vi "Get Discovered Devices (SubVI).vi"(8 "error in":errorcluster, 9 "DeviceKey List":string[](array[string]), 10 "Master Count":i32, 11 "CmdLib In":refnum<k24>) -> (0 "error out":errorcluster, 1 "DeviceKey List Out":string[](array[string]), 2 "Device Array":T1(array[cluster]), 3 "CmdLib Out":refnum<k24>)   [LabVIEW 2017]
doc: "by Tanguy BOULARD"
uses:
  dll/CmdLib.dll
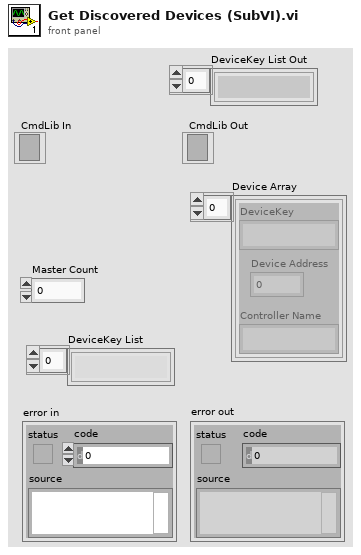
[diagram p1: front panel]
types:
  T1 = cluster{"DeviceKey":string, "Device Address":i32, "Controller Name":string}[]
  T2 = cluster{"DeviceKey Out":string, "Device Address Out":i32, "Controller Name":string}
  T3 = cluster{"DeviceKey Out":string, "Device Address Out":i32, "Controller Name":string}[]
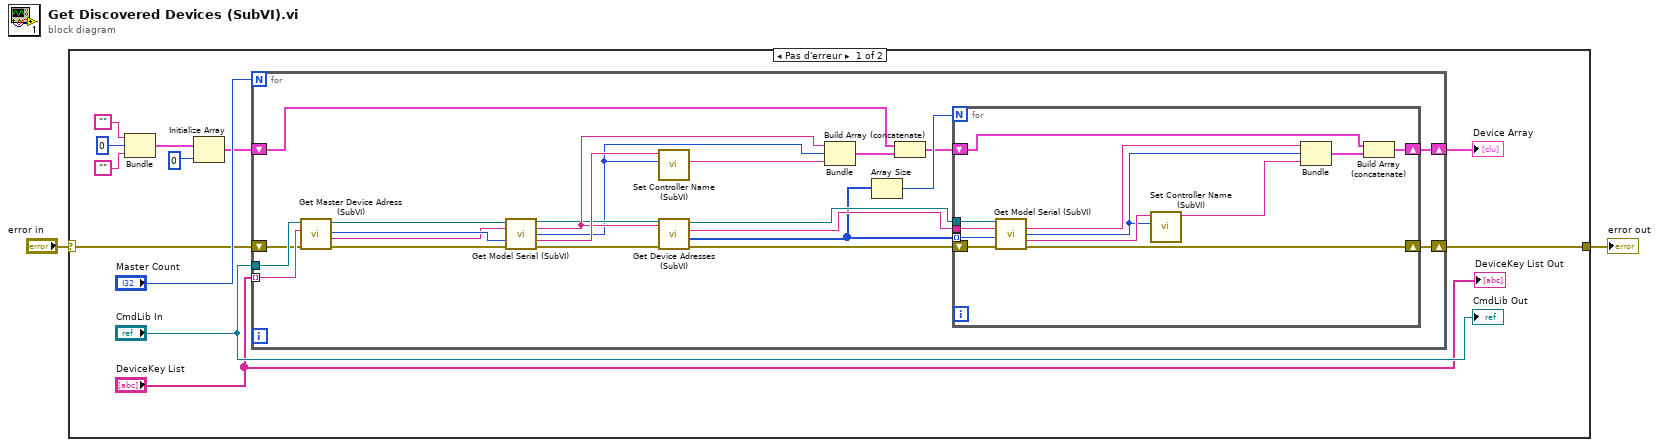
[diagram p0: block diagram]
diagram:
  n1 = case shown="Pas d'erreur" "error in" {
    selector: "error in" -> [w10 w50]
    tunnel: [w11 w50] -> w2
    frame No Error {
      n2 = Bundle("", 0, "") -> (w6:cluster{string, i32, string})  [unwired: 1 in]
      n3 = Initialize Array(w6, 0 ("dimension size")) -> (w4:cluster{string, i32, string}[])
      n4 = for {
        N: "Master Count" -> [_]
        tunnel: "CmdLib In" -> [w29]
        tunnel: "DeviceKey List" -> [w28] mode=indexing
        shift-right: [w26] -> w11
        shift-left: w10 -> [w27]
        shift-right: [w20] -> w3
        shift-left: w4 -> [w23]
        n5 = call "Get Master Device Adress (SubVI).vi"("entrée d'erreur (pas d'erreur)"=w27, "DeviceKey In"=w28, "Refnum de .NET en entrée"=w29) -> ("sortie d'erreur"=w36:errorcluster, "DeviceKey Out"=w24:string, "Device Address"=w25:i32, "Refnum de .NET en sortie"=w37:refnum<k24>)  [unwired: 5 in]
        n6 = call "Get Model Serial (SubVI).vi"("CmdLib In"=w37, "DeviceKey In"=w24, "Device Address In"=w25, "error in (no error)"=w36) -> ("CmdLib Out"=w16:refnum<k24>, "DeviceKey Out"=w17:string, "Device Address Out"=w15:i32, "Model / Serial"=w18:string, "error out"=w35:errorcluster)  [unwired: 7 in]
        n7 = call "Set Controller Name (SubVI).vi"("Device Address"=w15, "Model / Serial"=w18) -> ("Controller Name"=w19:string)  [unwired: 9 in]
        n8 = call "Get Device Adresses (SubVI).vi"("error in (no error)"=w35, "DeviceKey In"=w17, "CmdLib In"=w16) -> ("error out"=w31:errorcluster, "Device Addresses"=w30:i32[], "DeviceKey Out"=w33:string, "CmdLib Out"=w32:refnum<k24>)  [unwired: 5 in]
        n9 = Bundle("DeviceKey Out"=w17, "Device Address Out"=w15, "Controller Name"=w19) -> (w22:T2)  [unwired: 1 in]
        n10 = Array Size(array=w30) -> (size(s)=w34:i32)
        n11 = Build Array (concatenate)(w23, w22) -> (w21:T3)
        n12 = for {
          N: w34 -> [_]
          tunnel: w33 -> [w49]
          tunnel: w32 -> [w48]
          tunnel: w30 -> [w44] mode=indexing
          shift-right: [w47] -> w26
          shift-left: w31 -> [w45]
          shift-right: [w42] -> w20
          shift-left: w21 -> [w43]
          n13 = call "Get Model Serial (SubVI).vi"("CmdLib In"=w48, "DeviceKey In"=w49, "Device Address In"=w44, "error in (no error)"=w45) -> ("DeviceKey Out"=w38:string, "Device Address Out"=w39:i32, "Model / Serial"=w46:string, "error out"=w47:errorcluster)  [unwired: 7 in, 1 out]
          n14 = call "Set Controller Name (SubVI).vi"("Device Address"=w39, "Model / Serial"=w46) -> ("Controller Name"=w40:string)  [unwired: 9 in]
          n15 = Bundle("DeviceKey Out"=w38, "Device Address Out"=w39, "Controller Name"=w40) -> (w41:T2)  [unwired: 1 in]
          n16 = Build Array (concatenate)(w43, w41) -> (w42:T3)
        }
      }
      "Device Array" <- w3
      "CmdLib Out" <- "CmdLib In"
      "DeviceKey List Out" <- "DeviceKey List"
    }
    frame Error {
    }
  }
  "error out" <- w2
